vi "Data Viewer.vi"(8 "error in (no error)":errorcluster, 10 "Starting Waveforms":waveform(dbl)[](array[waveform])) -> (0 "error out":errorcluster, 3 "Data Viewer out":refnum<class "Logging.lvclass">)   [LabVIEW 2020, in "Logging.lvlib" / "Logging.lvclass"]
doc: "Initializes the Data Viewer Panel Actor.\n----\nCopyright: MGI 2017\nAuthor: Derek Trepanier"
uses:
  Logging.lvclass
  Logging.lvclass/Logging.ctl
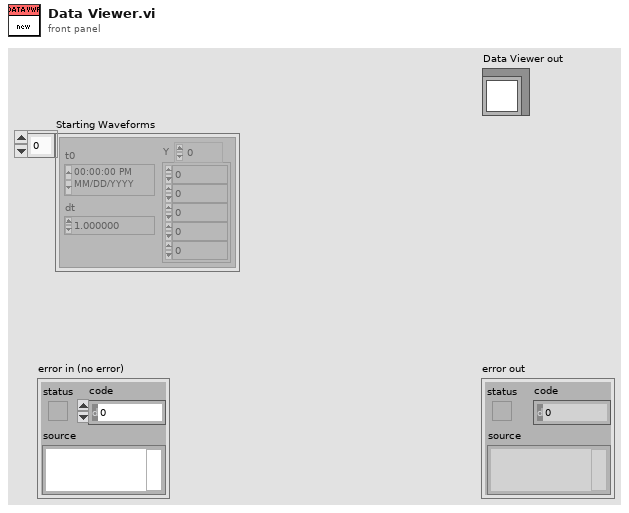
[diagram p1: front panel]
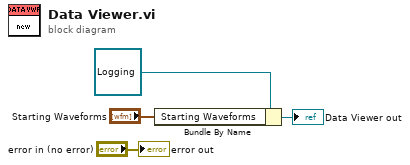
[diagram p0: block diagram]
diagram:
  n1 = Bundle By Name(cluster=refnum<class "Logging.lvclass"> refnum ("Data Viewer in"), "Starting Waveforms"="Starting Waveforms") -> (→"Data Viewer out":refnum<class "Logging.lvclass">)
  "error out" <- "error in (no error)"
